vi "Generate txt Report.vi"(0 "Serial Number":string, 1 "Testing result":string, 2 "Failed Tests":string, 3 "Upper Limits":dbl[](array[numeric]), 4 "Lower Limits":dbl[](array[numeric]), 5 "Measurement values":dbl[](array[numeric]), 6 "Test Names":string[](array[string]), 7 "Status":string[](array[string]), 9 "NTC Codes":string) -> (19 "error out":errorcluster)   [LabVIEW 2023]
uses:
  <vilib>/Utility/file.llb/Read Delimited Spreadsheet (string).vi
  <vilib>/Utility/file.llb/Write Delimited Spreadsheet (string).vi
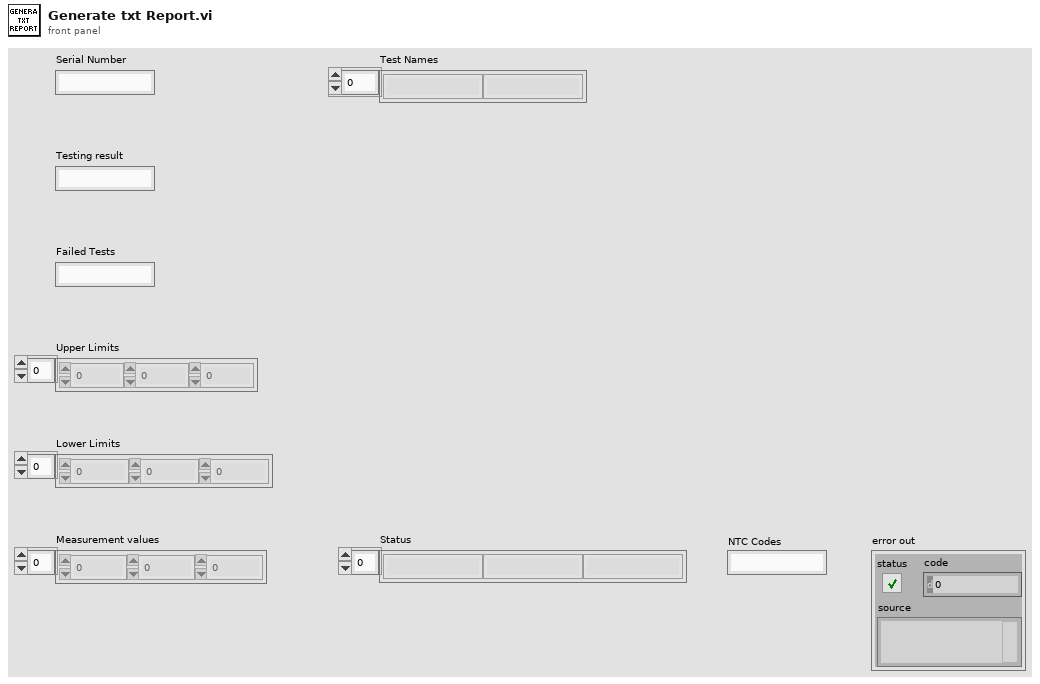
[diagram p1: front panel]
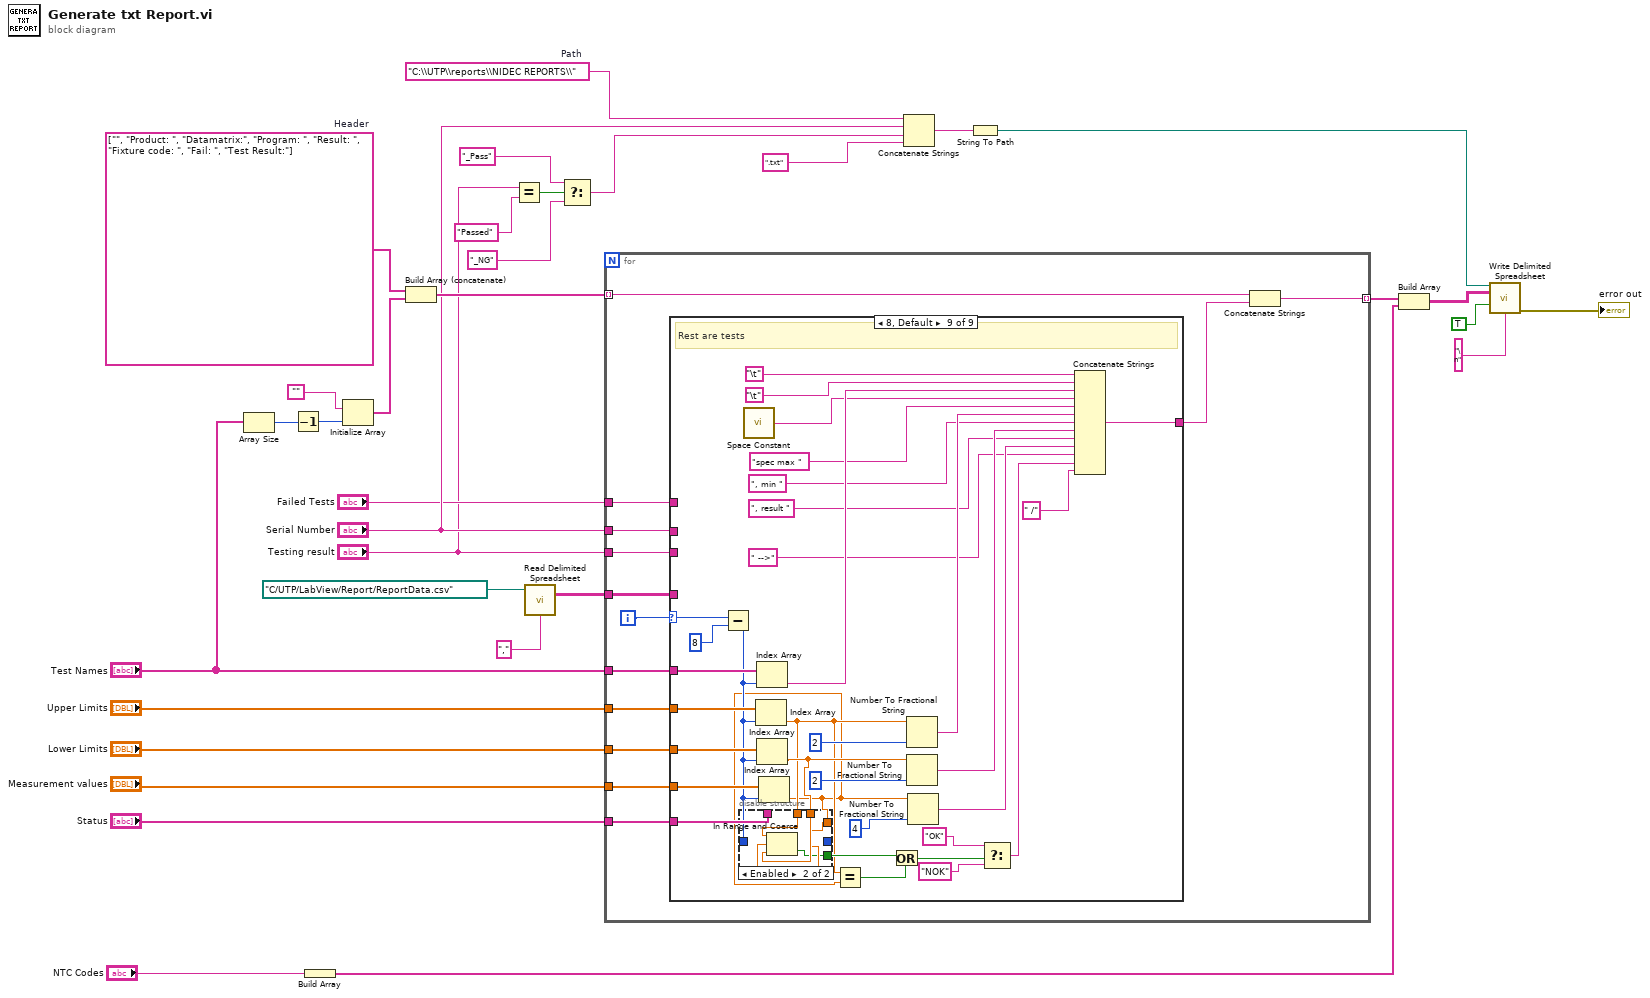
[diagram p0: block diagram]
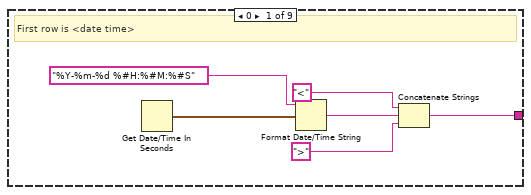
[diagram p2: hidden frame]
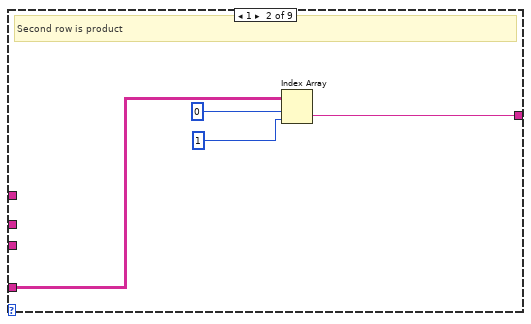
[diagram p3: hidden frame]
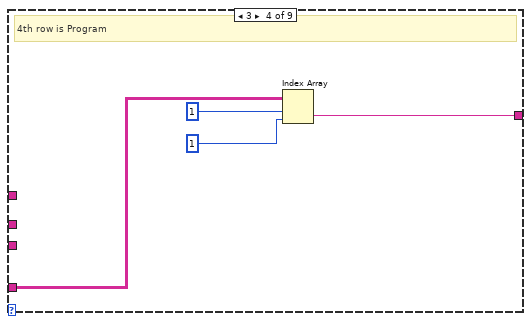
[diagram p5: hidden frame]
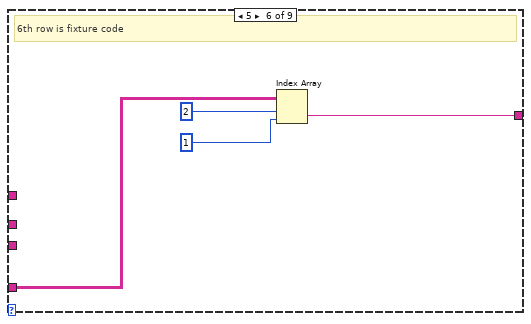
[diagram p7: hidden frame]
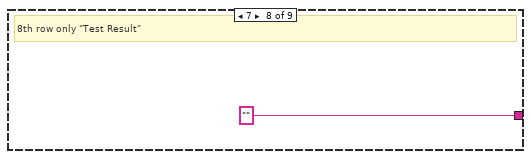
[diagram p9: hidden frame]
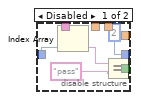
[diagram p10: hidden frame]
diagram:
  w28 = "C:\\UTP\\reports\\NIDEC REPORTS\\"  # Path
  w19 = string[] ["", "Product: ", "Datamatrix:", "Program: ", "Result: ", "Fixture code: ", "Fail: ", "Test Result:"]  # Header
  n1 = Array Size(array="Test Names") -> (size(s)=w22:i32)
  n2 = Decrement(x=w22) -> (x-1=w5:i32)
  n3 = Build Array("NTC Codes") -> (w1:string[])
  n4 = Initialize Array("", w5) -> (w20:string[])
  n5 = Build Array (concatenate)(w19, w20) -> (w16:string[])
  n6 = Equal?(x="Testing result", y="Passed") -> (x = y?=w10:bool)
  n7 = call-poly <vilib>:"Read Delimited Spreadsheet.vi"("file path (dialog if empty)"=path "C:/UTP/LabView/Report/ReportData.csv", "delimiter (\\t)"="," ("delimiter (\\t)")) -> ("all rows"=w15:string[][])  [unwired: 8 in, 5 out]
  n8 = Select(t="_Pass" ("y"), s=w10, f="_NG") -> (s? t:f=w7:string)
  n9 = for {
    tunnel: "Upper Limits" -> [w41]
    tunnel: "Lower Limits" -> [w40]
    tunnel: "Measurement values" -> [w39]
    tunnel: "Status" -> [w38]
    tunnel: "Test Names" -> [w42]
    tunnel: w16 -> [w36] mode=indexing
    tunnel: [w34] -> w4 mode=indexing
    tunnel: w15 -> [w45]
    tunnel: "Serial Number" -> [w44]
    tunnel: "Testing result" -> [w43]
    tunnel: "Failed Tests" -> [w37]
    i -> [w46]
    n10 = case shown="8, Default" w46 {
      selector: w46 -> [_ _ _ _ _ _ _ _ w96]
      tunnel: [w47 w53 w57 w58 w62 w63 w67 "" ("Failed Tests") w77] -> w35
      tunnel: w45 -> [_ w56 _ w59 _ w64 _ _ _]
      tunnel: w44 -> [_ _ w57 _ _ _ _ _ _]
      tunnel: w43 -> [_ _ _ _ w62 _ _ _ _]
      tunnel: w42 -> [_ _ _ _ _ _ _ _ w101]
      tunnel: w41 -> [_ _ _ _ _ _ _ _ w100]
      tunnel: w40 -> [_ _ _ _ _ _ _ _ w99]
      tunnel: w39 -> [_ _ _ _ _ _ _ _ w98]
      tunnel: w38 -> [_ _ _ _ _ _ _ _ w97]
      tunnel: w37 -> [_ _ _ _ _ _ w67 _ _]
      frame 0 {
        # "First row is <date time>"
        n11 = Get Date/Time In Seconds() -> (seconds since 1Jan1904=w52:timestamp)
        n12 = Format Date/Time String(time format string (%c)="%Y-%m-%d %#H:%#M:%#S", seconds (now)=w52) -> (date/time string=w51:string)  [unwired: 1 in]
        n13 = Concatenate Strings("<" ("string"), w51, ">" ("string")) -> (w47:string)
      }
      frame 1 {
        # "Second row is product"
        n14 = Index Array(array=w56, index (row)=0, index (col)=1) -> (element=w53:string)
      }
      frame 2 {
        # "third row is Datamatrix (Serial number)"
      }
      frame 3 {
        # "4th row is Program"
        n15 = Index Array(array=w59, index (row)=1, index (col)=1) -> (element=w58:string)
      }
      frame 4 {
        # "5th row is Overall testing result"
      }
      frame 5 {
        # "6th row is fixture code"
        n16 = Index Array(array=w64, index (row)=2, index (col)=1) -> (element=w63:string)
      }
      frame 6 {
        # "7th row is failed tests"
      }
      frame 7 {
        # "8th row only \"Test Result\""
      }
      frame 8, Default {
        # "Rest are tests"
        n17 = Subtract(x=w96, y=8) -> (x-y=w94:i32)
        n18 = call <vilib>:"Space Constant.vi"() -> ("String"=w88:string)
        n19 = Index Array(array=w100, index=w94) -> (element=w73:dbl)
        n20 = Index Array(array=w101, index=w94) -> (element=w89:string)
        n21 = Index Array(array=w99, index=w94) -> (element=w75:dbl)
        n22 = Index Array(array=w98, index=w94) -> (element=w72:dbl)
        n23 = disable-structure shown="Enabled" {
          disable-tunnel: [i16 2 ("precision (6)") _] -> _
          disable-tunnel: w97 -> [w106 _]
          disable-tunnel: w94 -> [w105 _]
          disable-tunnel: [w102 w108] -> w74
          disable-tunnel: w73 -> [_ w111]
          disable-tunnel: w75 -> [_ w110]
          disable-tunnel: w72 -> [_ w109]
          frame Disabled {
            n24 = Index Array(array=w106, index=w105) -> (element=w104:string)
            n25 = Equal?(x=w104, y="pass") -> (x = y?=w102:bool)
          }
          frame Enabled {
            n26 = In Range and Coerce(upper limit=w111, x=w109, lower limit=w110) -> (In Range?=w108:bool)  [unwired: 1 out]
          }
        }
        n27 = Equal?(x=w73, y=w72) -> (x = y?=w71:bool)
        n28 = Or(x=w74, y=w71) -> (x .or. y?=w70:bool)
        n29 = Number To Fractional String(number=w73, precision (6)=i16 2) -> (F-format string=w86:string)  [unwired: 2 in]
        n30 = Number To Fractional String(number=w75, precision (6)=i16 2) -> (F-format string=w84:string)  [unwired: 2 in]
        n31 = Number To Fractional String(number=w72, precision (6)=i16 4) -> (F-format string=w82:string)  [unwired: 2 in]
        n32 = Select(t="OK" ("y"), s=w70, f="NOK" ("y")) -> (s? t:f=w78:string)
        n33 = Concatenate Strings("\t", "\t", w89, w88, "spec max " ("string"), w86, ", min " ("string"), w84, ", result " ("string"), w82, " -->" ("string"), w78, " /" ("string")) -> (w77:string)
      }
    }
    n34 = Concatenate Strings(w36, w35) -> (w34:string)
  }
  n35 = Concatenate Strings(w28, "Serial Number", w7, ".txt" ("string")) -> (w27:string)
  n36 = String To Path(string=w27) -> (path=w26:path)
  n37 = Build Array(w4, w1) -> (w3:string[][])
  n38 = call-poly <vilib>:"Write Delimited Spreadsheet.vi"("file path (dialog if empty)"=w26, "2D data"=w3, "append to file? (new file:F)"=TRUE, "delimiter (\\t)"="\n" ("delimiter (\\t)")) -> ("error out"=→"error out":errorcluster)  [unwired: 10 in, 1 out]
